vi "Square Function.vi"(1 "x":dbl format="%0.2f") -> (0 "square(x)":dbl format="%0.2f")   [LabVIEW 2020, in "NI_Gmath.lvlib"]
doc: "Generates the square function for any real number <B>x</B>."
uses:
  <vilib>/gmath/NI_Gmath.lvlib
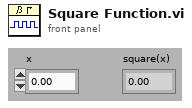
[diagram p1: front panel]
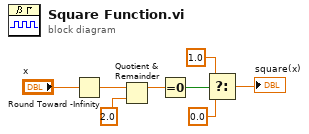
[diagram p0: block diagram]
diagram:
  n1 = Round Toward -Infinity(1:"x") -> (0:w2:dbl)
  n2 = Quotient & Remainder(x=w2, y=2.0) -> (x-y*floor(x/y)=w7:dbl)  [unwired: 1 out]
  n3 = Equal To 0?(x=w7) -> (x = 0?=w8:bool)
  n4 = Select(t=1.0, s=w8, f=0.0) -> (s? t:f=→"square(x)":dbl)
